vi "Calculate Position.vi"(11 "Drive HW Status":T1) -> (2 "Reset":bool, 3 "Distance":dbl format="%0.2f", 5 "Distances":dbl[](array[numeric]))   [LabVIEW 2017, in "MechamunDrive.lvlib"]
uses:
  MechamunDrive.lvlib
  Cluster_HW Status.ctl
  TypeDefs/Cluster_SRX Status With Encoder.ctl
panel:
  in  "Encoder to Wheel Rotation":dbl=2.0
  in  "CPR":dbl=2048.0
  in  "Wheel Size(in)":dbl=8.0
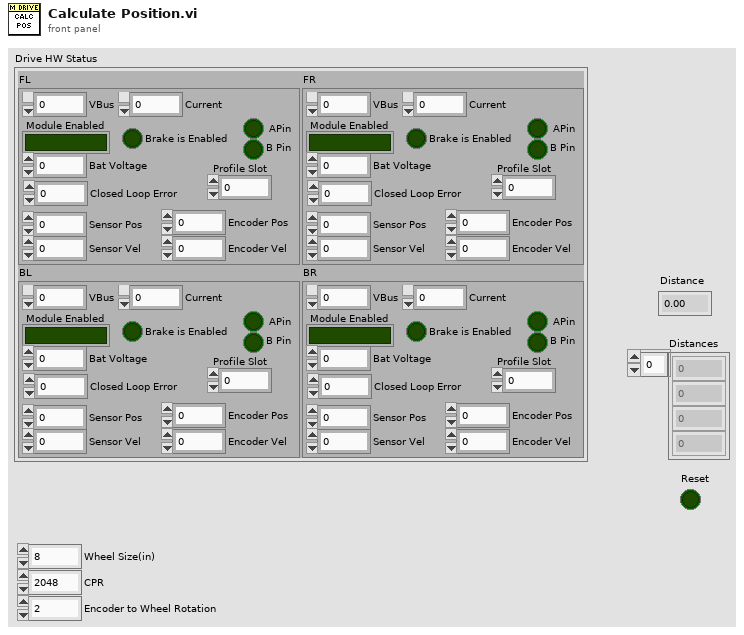
[diagram p1: front panel]
types:
  T1 = typedef "MechamunDrive.lvlib/Cluster_HW Status.ctl" = cluster{"BL":T2, "BR":T2, "FL":T2, "FR":T2}
  T2 = typedef "Cluster_SRX Status With Encoder.ctl" = cluster{"VBus ":dbl, "Module Enabled":bool, "Closed Loop Error":dbl, "Sensor Pos":dbl, "Sensor Vel":dbl, "Current":dbl, "Brake is Enabled":bool, "Encoder Pos":dbl, "Encoder Vel":dbl, " APin":bool, "B Pin":bool, "Bat Voltage":dbl, "Profile Slot":dbl}
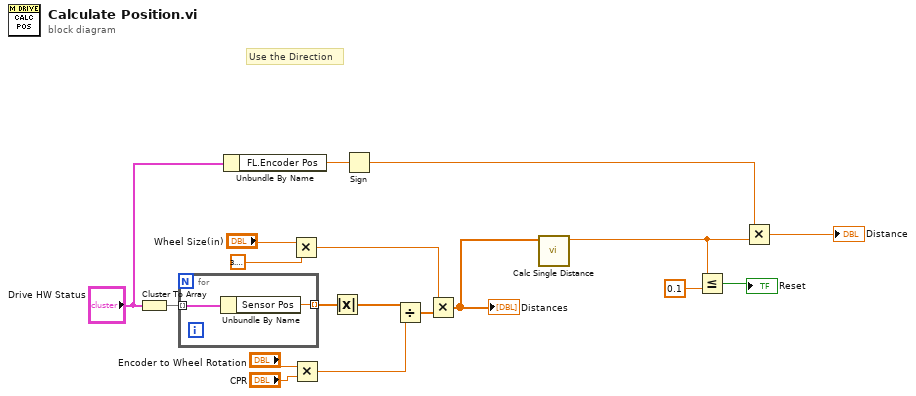
[diagram p0: block diagram]
diagram:
  # "Use the Direction"
  n1 = Cluster To Array(cluster="Drive HW Status") -> (array=w18:T2[])
  n2 = for {
    tunnel: w18 -> [w20] mode=indexing
    tunnel: [w19] -> w17 mode=indexing
    n3 = Unbundle By Name(w20) -> ("Sensor Pos"=w19:dbl)
  }
  n4 = Unbundle By Name("Drive HW Status") -> ("FL.Encoder Pos"=w3:dbl)
  n5 = Multiply(x="Wheel Size(in)", y=3.141592653589793) -> (x*y=w9:dbl)
  n6 = Multiply(x="Encoder to Wheel Rotation", y="CPR") -> (x*y=w11:dbl)
  n7 = Absolute Value(x=w17) -> (abs(x)=w12:dbl[])
  n8 = Sign(1:w3) -> (0:w1:dbl)
  n9 = Divide(x=w12, y=w11) -> (x/y=w10:dbl[])
  n10 = Multiply(x=w9, y=w10) -> (x*y=w8:dbl[])
  "Distances" <- w8
  n11 = call "Calc Single Distance.vi"("Drive Position Array"=w8) -> ("mean"=w7:dbl)  [unwired: 10 in]
  n12 = Less Or Equal?(x=w7, y=0.1) -> (x <= y?=→"Reset":bool)
  n13 = Multiply(x=w1, y=w7) -> (x*y=→"Distance":dbl)
